vi "Illini Hyperloop GUI v3.vi"() -> ()   [LabVIEW 2015]
uses:
  <vilib>/robotics/Controls/Attitude Indicator/Attitude Indicator.xctl
  CommunicationStatus.ctl
  StageEnum.ctl
  BlockDiagramControlEnum.ctl
  <vilib>/ErrorRing/Error Ring.xnode
panel:
  out "Braking Force":dbl
  out "Braking Force Chart":dbl(slide) caption="Braking Force (N)" scale=0.0..10000.0
  out "Current 6":dbl[unit] caption="Current"
  out "Voltage 6":dbl[unit] caption="Voltage"
  out "RPM 6":dbl[unit] caption="RPM"
  out "Current 5":dbl[unit] caption="Current"
  out "Voltage 5":dbl[unit] caption="Voltage"
  out "RPM 5":dbl[unit] caption="RPM"
  out "Current 4":dbl[unit] caption="Current"
  out "Voltage 4":dbl[unit] caption="Voltage"
  out "RPM 4":dbl[unit] caption="RPM"
  out "Current 3":dbl[unit] caption="Current"
  out "Voltage 3":dbl[unit] caption="Voltage"
  out "RPM 3":dbl[unit] caption="RPM"
  out "Current 2":dbl[unit] caption="Current"
  out "Voltage 2":dbl[unit] caption="Voltage"
  out "RPM 2":dbl[unit] caption="RPM"
  out "Current 1":dbl[unit] caption="Current"
  out "Voltage 1":dbl[unit] caption="Voltage"
  out "RPM 1":dbl[unit] caption="RPM"
  out "Flight Time":string
  out "Attitude Indicator":cluster{"Roll":dbl, "Pitch":dbl}(xcontrol)
  out "Yaw":dbl(knob) scale=-20.0..20.0
  out "RPM Gauge 6":dbl(knob) scale=0.0..2000.0
  out "RPM Gauge 5":dbl(knob) scale=0.0..2000.0
  out "RPM Gauge 4":dbl(knob) scale=0.0..2000.0
  out "RPM Gauge 3":dbl(knob) scale=0.0..2000.0
  out "RPM Gauge 2":dbl(knob) scale=0.0..2000.0
  out "RPM Gauge 1":dbl(knob) scale=0.0..2000.0
  out "Cabin Pressure":dbl format="%#.3g"
  out "Cabin Pressure (psi)":dbl(graph)
  out "Stage":T1
  out "Communication Status":T2
  out "Levitation Height":dbl[unit]
  out "Computing:":dbl format="%#.2g"
  out "Low Battery":dbl format="%#.2g"
  out "High Battery:":dbl format="%#.2g"
  out "Battery 3":dbl(slide) scale=0.0..100.0
  out "Battery 2":dbl(slide) scale=0.0..100.0
  out "Battery 1":dbl(slide) scale=0.0..100.0
  out "Z acceleration":dbl
  out "Y acceleration":dbl
  out "X acceleration":dbl
  out "Z velocity":dbl
  out "Y velocity":dbl
  out "X velocity":dbl
  out "Z position":dbl
  out "Y position":dbl
  out "X position":dbl
  out "Position (m)":dbl(slide) scale=0.0..2490.0
  out "Checkmark":u16(ring)
  out "Velocity (m/s)":dbl(graph)
  in  "EMERGENCY BRAKE":bool
  in  "Functional Test Tab Control":T3(tab)
  out "Functional Test A Data":string caption="Data:"
  in  "Functional Test 1":bool caption="Boolean"
  out "Functional Test B Data":string caption="Data:"
  in  "Functional Test 2":bool caption="Boolean"
  out "Functional Test C Data":string caption="Data:"
  in  "Functional Test 3":bool caption="Boolean"
  in  "Functional Test 4":bool caption="Boolean"
  out "Functional Test D Data":string caption="Data:"
  in  "Client Closed":string="The client VI closed the connection."
  out "Data out":string
  out "remote address":string
  out "remote port":u16
  in  "Prepare for Launch":bool caption="Boolean"
  in  "Stop Program":bool
  out "Temp 2:":dbl format="%.2g"
  out "Temp 1:":dbl format="%.2g"
  out "Temperature (K)":dbl[](graph)
  out "Acceleration Chart":dbl(graph)
  # "Illini Hyperloop"
  # "Arx Pax"
  # "Front"
  # "Attitude"
  # "Acceleration (m/s/s)"
  # "Battery Levels (%)"
  # "More battery?????"
  # "Functional Test A: Power Up and Communication"
  # "Functional Test B: Levitation"
  # "Functional Test C: Communication Inside Tube"
  # "Functional Test D: Internal power and Levitation"
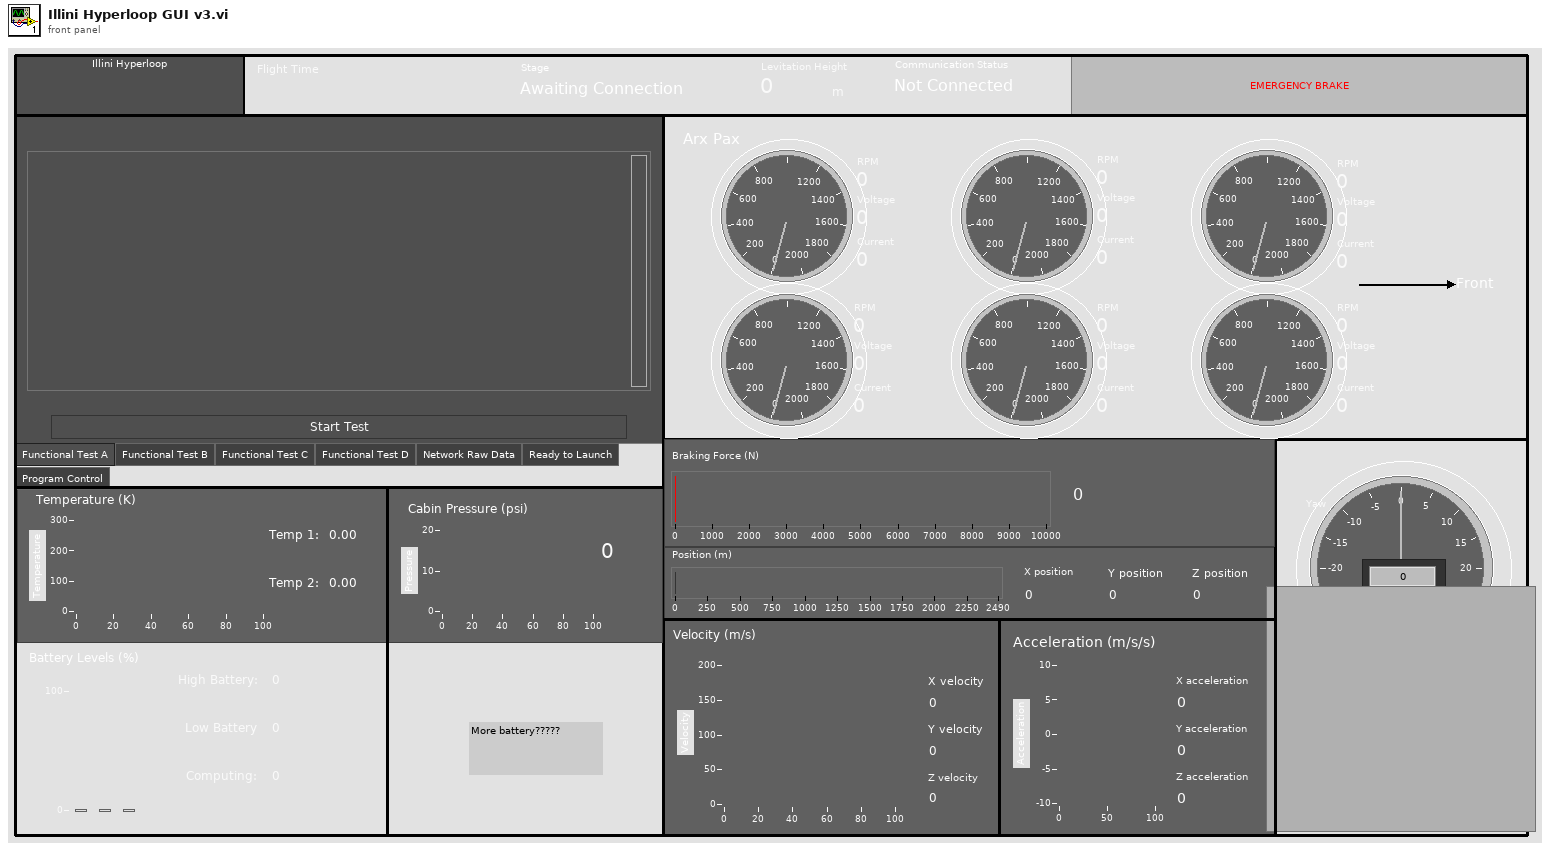
[diagram p1: front panel]
types:
  T1 = typedef "StageEnum.ctl" = enum16{"Awaiting Connection", "TEST Comms", "TEST Lev", "TEST Inside Comms", "TEST Internal Power", "Ready to Launch", "Acceleration", "Coast", "Brake"}
  T2 = typedef "CommunicationStatus.ctl" = enum16{"Not Connected", "Connected", "Disconnected"}
  T3 = enum32{"Functional Test A", "Functional Test B", "Functional Test C", "Functional Test D", "Network Raw Data", "Ready to Launch", "Program Control"}
  T4 = typedef "BlockDiagramControlEnum.ctl" = enum16{"Not Connected", "Disconnected", "Functional Test A", "Functional Test B", "Functional Test C", "Functional Test D", "Flight"}
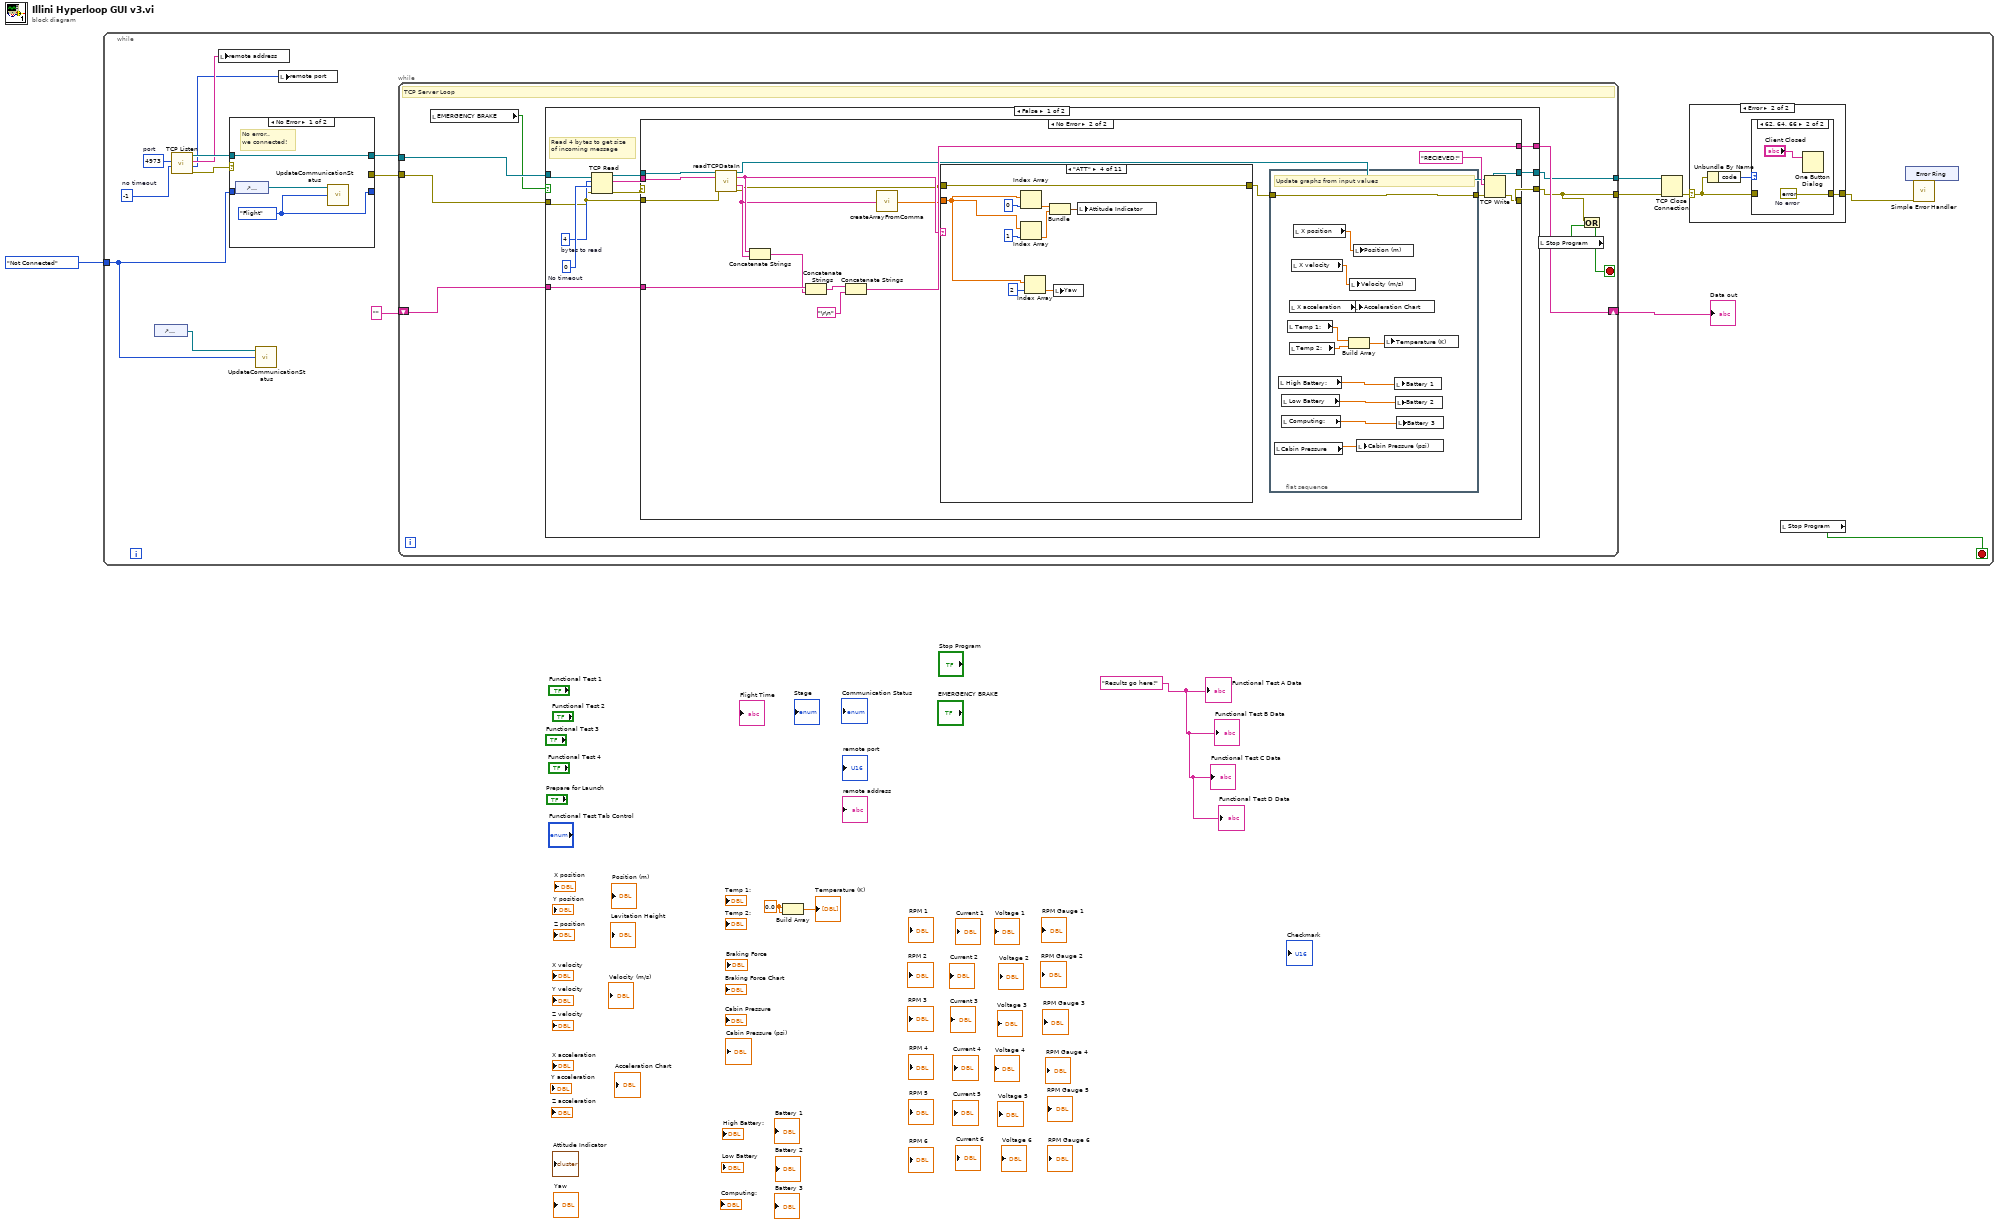
[diagram p0: block diagram]
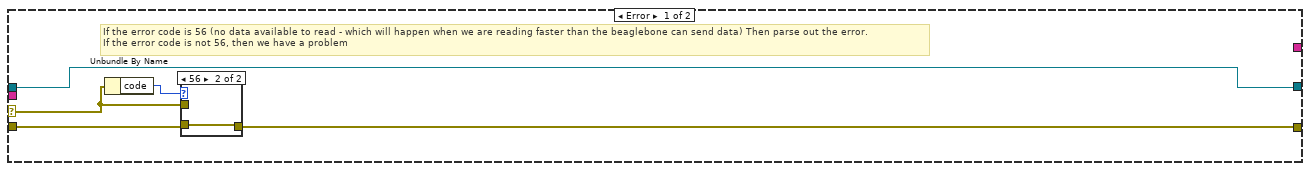
[diagram p5: hidden frame]
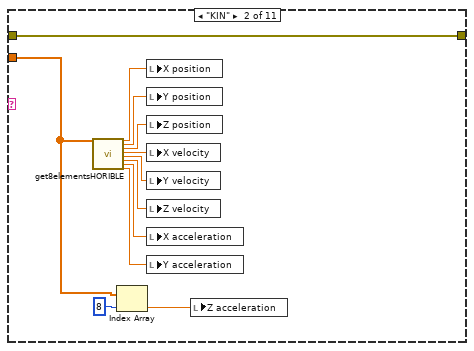
[diagram p8: hidden frame]
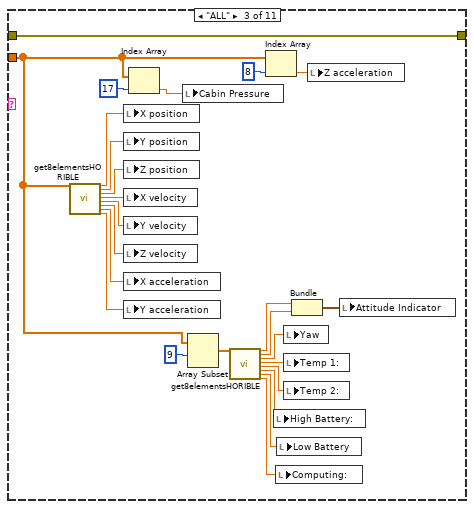
[diagram p9: hidden frame]
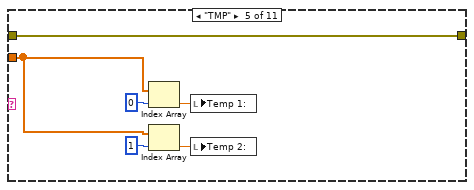
[diagram p10: hidden frame]
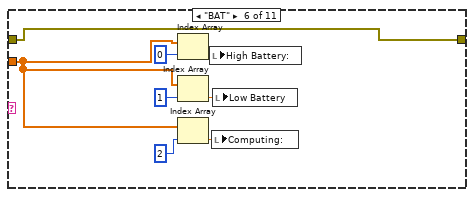
[diagram p11: hidden frame]
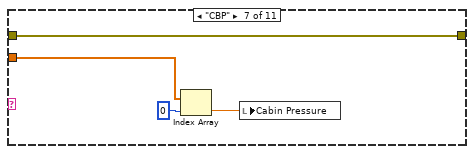
[diagram p12: hidden frame]
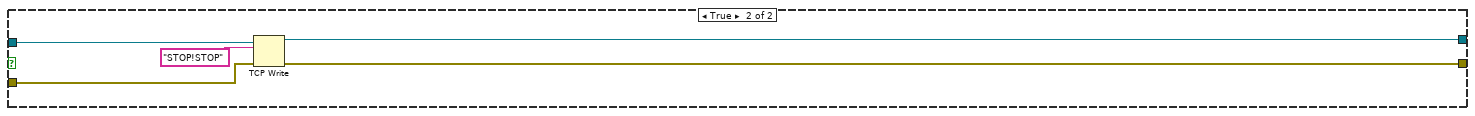
[diagram p17: hidden frame]
diagram:
  w2 = 0.0 ("element")
  w4 = "Results go here!" ("Functional Test 1 Data")
  n1 = while {
    tunnel: BlockDiagramControlEnum."Not Connected" -> [w5]
    stop <- w13 stop-if-true
    w18 = u16 4973  # port
    w19 = -1  # no timeout
    n2 = control-ref of="Communication Status"() -> (w6:refnum<vi>)
    n3 = call <vilib>:"TCP Listen.vi"("timeout ms (wait forever: -1)"=w19, "port"=w18) -> ("error out"=w10:errorcluster, "remote port"=w7:u16, "remote address"=w8:string, "connection ID"=w12:refnum<k5>)  [unwired: 5 in, 1 out]
    n4 = local write "remote address"(w8) -> ()
    n5 = case shown="No Error" w10 {
      selector: w10 -> [_ w26]
      tunnel: w12 -> [w24 w27]
      tunnel: [w24 w27] -> w11
      tunnel: [_ w26] -> w9
      tunnel: w5 -> [_ w25]
      tunnel: [w22 w25] -> _
      frame No Error {
        w22 = BlockDiagramControlEnum."Flight"
        # "No error.. \nwe connected!"
        n6 = control-ref of="Communication Status"() -> (w23:refnum<vi>)
        n7 = call "UpdateCommunicationStatus.vi"("Block Diagram Control Enum"=w22, "Communication Enum Refnum in"=w23) -> ()  [unwired: 1 in]
      }
      frame Error {
      }
    }
    n8 = call "UpdateCommunicationStatus.vi"("Block Diagram Control Enum"=w5, "Communication Enum Refnum in"=w6) -> ()  [unwired: 1 in]
    n9 = local write "remote port"(w7) -> ()
    n10 = while {
      tunnel: w11 -> [w43]
      tunnel: w9 -> [w44]
      shift-right: [w41] -> w16
      shift-left: "" -> [w42]
      tunnel: [w40] -> w15
      tunnel: [w37] -> w14
      stop <- w36 stop-if-true
      # "TCP Server Loop"
      n11 = local read "EMERGENCY BRAKE"() -> (w39:bool)
      n12 = case shown="False" w39 {
        tunnel: w44 -> [w53 w165]
        tunnel: w43 -> [w54 w164]
        tunnel: [w49 w163] -> w40
        tunnel: [w51 w162] -> w37
        tunnel: w42 -> [w47 _]
        tunnel: [w46 _] -> w41
        frame False {
          w55 = 4  # bytes to read
          w56 = 0  # No timeout
          # "Read 4 bytes to get size\nof incoming message"
          n13 = TCP Read(connection ID=w54, bytes to read=w55, error in (no error)=w53, 9:w56) -> (connection ID out=w50:refnum<k5>, data out=w48:string, error out=w52:errorcluster)  [unwired: 1 in]
          n14 = case shown="No Error" w52 {
            selector: w52 -> [w59 _]
            tunnel: w53 -> [w60 w79]
            tunnel: [w58 w64] -> w51
            tunnel: w50 -> [w57 w80]
            tunnel: [w57 w66] -> w49
            tunnel: w48 -> [_ w81]
            tunnel: w47 -> [_ w78]
            tunnel: [_ w74] -> w46
            frame Error {
              # "If the error code is 56 (no data available to read - which will happen when we are reading faster than the beaglebone can send data) Then parse out the error. \nIf the error code is not 56, then we have a problem"
              n15 = Unbundle By Name(w59) -> ("code"=w61:i32)
              n16 = case shown="56" w61 {
                tunnel: w59 -> [w62 _]
                tunnel: [w62 w63] -> w58
                tunnel: w60 -> [_ w63]
                frame Default {
                }
                frame 56 {
                }
              }
            }
            frame No Error {
              n17 = call "readTCPDataIn.vi"("TCP Network Connection in"=w80, "Size of data"=w81, "error in (no error)"=w79) -> ("TCP Network Connection out"=w67:refnum<k5>, "Operation"=w73:string, "Data"=w71:string, "error out"=w69:errorcluster)  [unwired: 8 in, 1 out]
              n18 = Concatenate Strings(w73, w71) -> (w72:string)
              n19 = Concatenate Strings(w78, w72) -> (w75:string)
              n20 = Concatenate Strings(w75, "\r\n") -> (w74:string)
              n21 = call "createArrayFromComma.vi"("String"=w71) -> ("Array"=w70:dbl[])
              n22 = case shown="\"ATT\"" w73 {
                tunnel: w70 -> [_ w104 w108 w136 w143 w150 w156 _ _ _ _]
                tunnel: w69 -> [w93 w102 w106 w131 w140 w146 w154 w158 w159 w160 w161]
                tunnel: [w93 w102 w106 w131 w140 w146 w154 w158 w159 w160 w161] -> w77
                frame Default {
                }
                frame "KIN" {
                  n23 = call "get8elementsHORIBLE.vi"("Array"=w104) -> ("Numeric"=w101:dbl, "Numeric 2"=w100:dbl, "Numeric 3"=w99:dbl, "Numeric 4"=w98:dbl, "Numeric 5"=w97:dbl, "Numeric 6"=w96:dbl, "Numeric 7"=w95:dbl, "Numeric 8"=w94:dbl)  [unwired: 19 in]
                  n24 = Index Array(array=w104, index=8) -> (element=w103:dbl)
                  n25 = local write "X position"(w101) -> ()
                  n26 = local write "Y position"(w100) -> ()
                  n27 = local write "Z position"(w99) -> ()
                  n28 = local write "X velocity"(w98) -> ()
                  n29 = local write "Y velocity"(w97) -> ()
                  n30 = local write "Z velocity"(w96) -> ()
                  n31 = local write "X acceleration"(w95) -> ()
                  n32 = local write "Y acceleration"(w94) -> ()
                  n33 = local write "Z acceleration"(w103) -> ()
                }
                frame "ALL" {
                  n34 = call "get8elementsHORIBLE.vi"("Array"=w108) -> ("Numeric"=w128:dbl, "Numeric 2"=w127:dbl, "Numeric 3"=w126:dbl, "Numeric 4"=w125:dbl, "Numeric 5"=w124:dbl, "Numeric 6"=w123:dbl, "Numeric 7"=w122:dbl, "Numeric 8"=w121:dbl)  [unwired: 19 in]
                  n35 = local write "X position"(w128) -> ()
                  n36 = local write "Y position"(w127) -> ()
                  n37 = local write "Z position"(w126) -> ()
                  n38 = local write "X velocity"(w125) -> ()
                  n39 = local write "Y velocity"(w124) -> ()
                  n40 = local write "Z velocity"(w123) -> ()
                  n41 = local write "X acceleration"(w122) -> ()
                  n42 = local write "Y acceleration"(w121) -> ()
                  n43 = Index Array(array=w108, index=17) -> (element=w107:dbl)
                  n44 = local write "Cabin Pressure"(w107) -> ()
                  n45 = Array Subset(array=w108, index=9) -> (w118:dbl[])  [unwired: 1 in]
                  n46 = call "get8elementsHORIBLE.vi"("Array"=w118) -> ("Numeric"=w117:dbl, "Numeric 2"=w116:dbl, "Numeric 3"=w115:dbl, "Numeric 4"=w114:dbl, "Numeric 5"=w113:dbl, "Numeric 6"=w112:dbl, "Numeric 7"=w111:dbl, "Numeric 8"=w110:dbl)  [unwired: 19 in]
                  n47 = Index Array(array=w108, index=8) -> (element=w129:dbl)
                  n48 = local write "High Battery:"(w112) -> ()
                  n49 = local write "Computing:"(w110) -> ()
                  n50 = local write "Low Battery"(w111) -> ()
                  n51 = local write "Yaw"(w115) -> ()
                  n52 = local write "Temp 1:"(w114) -> ()
                  n53 = local write "Temp 2:"(w113) -> ()
                  n54 = Bundle("Numeric"=w117, "Numeric 2"=w116) -> (w120:cluster{"Numeric":dbl, "Numeric 2":dbl})  [unwired: 1 in]
                  n55 = local write "Z acceleration"(w129) -> ()
                  n56 = local write "Attitude Indicator"(w120) -> ()
                }
                frame "ATT" {
                  n57 = Index Array(array=w136, index=0) -> (element=w135:dbl)
                  n58 = Index Array(array=w136, index=1) -> (element=w134:dbl)
                  n59 = Index Array(array=w136, index=2) -> (element=w132:dbl)
                  n60 = Bundle(w135, w134) -> (w133:cluster{dbl, dbl})  [unwired: 1 in]
                  n61 = local write "Yaw"(w132) -> ()
                  n62 = local write "Attitude Indicator"(w133) -> ()
                }
                frame "TMP" {
                  n63 = Index Array(array=w143, index=0) -> (element=w142:dbl)
                  n64 = Index Array(array=w143, index=1) -> (element=w141:dbl)
                  n65 = local write "Temp 1:"(w142) -> ()
                  n66 = local write "Temp 2:"(w141) -> ()
                }
                frame "BAT" {
                  n67 = Index Array(array=w150, index=0) -> (element=w149:dbl)
                  n68 = Index Array(array=w150, index=1) -> (element=w148:dbl)
                  n69 = Index Array(array=w150, index=2) -> (element=w147:dbl)
                  n70 = local write "High Battery:"(w149) -> ()
                  n71 = local write "Computing:"(w147) -> ()
                  n72 = local write "Low Battery"(w148) -> ()
                }
                frame "CBP" {
                  n73 = Index Array(array=w156, index=0) -> (element=w155:dbl)
                  n74 = local write "Cabin Pressure"(w155) -> ()
                }
                frame "FTA" {
                }
                frame "FTB" {
                }
                frame "FCC" {
                }
                frame "FCD" {
                }
              }
              n75 = flat-sequence {
                tunnel: w77 -> [w89]
                tunnel: [w89] -> w65
                frame #0 {
                  # "Update graphs from input values"
                  n76 = local read "Cabin Pressure"() -> (w85:dbl)
                  n77 = local read "High Battery:"() -> (w88:dbl)
                  n78 = local read "Low Battery"() -> (w87:dbl)
                  n79 = local read "Computing:"() -> (w86:dbl)
                  n80 = local read "Temp 1:"() -> (w84:dbl)
                  n81 = local read "Temp 2:"() -> (w83:dbl)
                  n82 = local read "X acceleration"() -> (w90:dbl)
                  n83 = local read "X velocity"() -> (w91:dbl)
                  n84 = local read "X position"() -> (w92:dbl)
                  n85 = Build Array(w84, w83) -> (w82:dbl[])
                  n86 = local write "Velocity (m/s)"(w91) -> ()
                  n87 = local write "Acceleration Chart"(w90) -> ()
                  n88 = local write "Position (m)"(w92) -> ()
                  n89 = local write "Cabin Pressure (psi)"(w85) -> ()
                  n90 = local write "Temperature (K)"(w82) -> ()
                  n91 = local write "Battery 1"(w88) -> ()
                  n92 = local write "Battery 2"(w87) -> ()
                  n93 = local write "Battery 3"(w86) -> ()
                }
              }
              n94 = TCP Write(connection ID=w67, data in="RECIEVED!", error in (no error)=w65) -> (connection ID out=w66:refnum<k5>, error out=w64:errorcluster)  [unwired: 1 in, 1 out]
            }
          }
        }
        frame True {
          n95 = TCP Write(connection ID=w164, data in="STOP!STOP", error in (no error)=w165) -> (connection ID out=w163:refnum<k5>, error out=w162:errorcluster)  [unwired: 1 in, 1 out]
        }
      }
      n96 = Wait (ms)(milliseconds to wait=u32 0) -> ()  [unwired: 1 out]
      n97 = local read "Stop Program"() -> (w38:bool)
      n98 = Or(x=w37, y=w38) -> (x .or. y?=w36:bool)
    }
    "Data out" <- w16
    n99 = TCP Close Connection(connection ID=w15, error in (no error)=w14) -> (error out=w21:errorcluster)  [unwired: 2 out]
    n100 = case shown="Error" w21 {
      selector: w21 -> [w29 w31]
      tunnel: [w29 w30] -> w20
      frame No Error {
      }
      frame Error {
        n101 = Unbundle By Name(w31) -> ("code"=w32:i32)
        n102 = case shown="62, 64, 66" w32 {
          tunnel: w31 -> [w33 _]
          tunnel: [w33 w35] -> w30
          frame Default {
          }
          frame 62, 64, 66 {
            w35 = errorcluster {"status"=FALSE, "code"=0, "source"=""}  # No error
            n103 = One Button Dialog(message="Client Closed") -> ()  [unwired: 1 in, 1 out]
          }
        }
      }
    }
    n104 = local read "Stop Program"() -> (w13:bool)
    n105 = xnode "Error Ring"() -> ()  [unwired: 1 out]
    n106 = call <vilib>:"Simple Error Handler.vi"("error in (no error)"=w20) -> ()  [unwired: 1 in, 8 out]
  }
  n107 = Build Array(w2, w2) -> (→"Temperature (K)":dbl[])
  "Functional Test A Data" <- w4
  "Functional Test B Data" <- w4
  "Functional Test C Data" <- w4
  "Functional Test D Data" <- w4
